vi "saveImage.vi"(9 "save_txt":bool, 10 "save_tiff":bool, 11 "image_info":T1={"file_path"=path "", "file_name"="", "image"=[], "image_size_xy"={"image_size_x_um"=1.0, "image_size_y_um"=1.0}, "pixel_dwell_time_ms"=1.0, "Laser_power_mW"=1.0, "pixel_size"=0.0, "tile_ij"={"tile_i"=0, "tile_j"=0}, "Objective"="", "ColorMarkers"=[], "timestamp"=timestamp(0 s since 1904-01-01), "micro-position-xyz"={"micro-position_x_mm"=1.0, "micro-position_y_mm"=1.0, "micro-position_z_mm"=1.0}, "zero_xyz"={"zero_x_mm"=0.0, "zero_y_mm"=0.0, "zero_z_mm"=0.0}, "nano-position-xyz"={"nano-position_x_V"=1.0, "nano-position_y_V"=1.0, "nano-position_z_V"=1.0}, "Kxyz"={"Kx_V/um"=1.0, "Ky_V/um"=1.0, "Kz_V/um"=1.0}}) -> ()   [LabVIEW 2018]
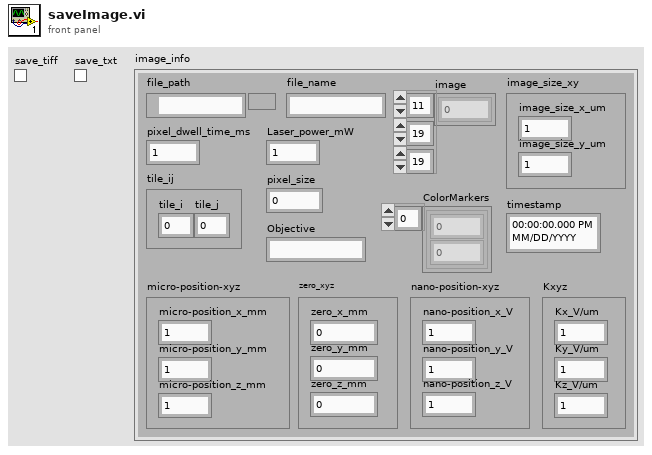
[diagram p1: front panel]
types:
  T1 = cluster{"file_path":path, "file_name":string, "image":dbl[][][], "image_size_xy":cluster{"image_size_x_um":sgl, "image_size_y_um":sgl}, "pixel_dwell_time_ms":sgl, "Laser_power_mW":sgl, "pixel_size":dbl, "tile_ij":cluster{"tile_i":i32, "tile_j":i32}, "Objective":string, "ColorMarkers":cluster{dbl, u32}[], "timestamp":timestamp, "micro-position-xyz":cluster{"micro-position_x_mm":sgl, "micro-position_y_mm":sgl, "micro-position_z_mm":sgl}, "zero_xyz":cluster{"zero_x_mm":dbl, "zero_y_mm":dbl, "zero_z_mm":dbl}, "nano-position-xyz":cluster{"nano-position_x_V":sgl, "nano-position_y_V":sgl, "nano-position_z_V":sgl}, "Kxyz":cluster{"Kx_V/um":sgl, "Ky_V/um":sgl, "Kz_V/um":sgl}}
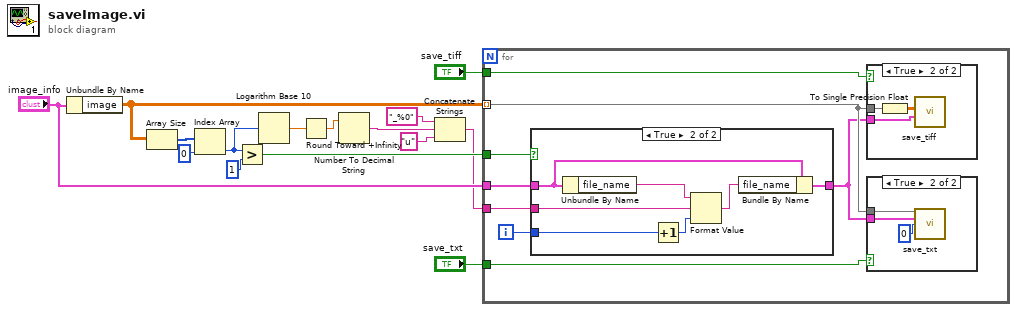
[diagram p0: block diagram]
diagram:
  n1 = Unbundle By Name("image_info") -> ("image"=w13:dbl[][][])
  n2 = Array Size(array=w13) -> (size(s)=w12:i32[])
  n3 = Index Array(array=w12, index=0) -> (element=w3:i32)
  n4 = Greater?(x=w3, y=1) -> (0:w9:bool)
  n5 = Logarithm Base 10(1:w3) -> (0:w2:dbl)
  n6 = Round Toward +Infinity(x=w2) -> (ceil(x): smallest int >= x=w1:dbl)
  n7 = Number To Decimal String(number=w1) -> (decimal integer string=w7:string)  [unwired: 1 in]
  n8 = Concatenate Strings("_%0" ("string"), w7, "u" ("string")) -> (w4:string)
  n9 = for {
    tunnel: "save_tiff" -> [w23]
    tunnel: "save_txt" -> [w22]
    tunnel: w13 -> [w21] mode=indexing
    tunnel: "image_info" -> [w18]
    tunnel: w9 -> [w20]
    tunnel: w4 -> [w16]
    i -> [w19]
    n10 = case shown="True" w20 {
      tunnel: w19 -> [_ w31]
      tunnel: w18 -> [w24 w26]
      tunnel: [w24 w28] -> w17
      tunnel: w16 -> [_ w25]
      frame False {
      }
      frame True {
        n11 = Unbundle By Name(w26) -> ("file_name"=w27:string)
        n12 = Increment(x=w31) -> (x+1=w30:i32)
        n13 = Format Value(string ("")=w27, format string=w25, value (0)=w30) -> (output string=w29:string)
        n14 = Bundle By Name(cluster=w26, "file_name"=w29) -> (w28:T1)
      }
    }
    n15 = case shown="True" w23 {
      tunnel: w21 -> [_ w35]
      tunnel: w17 -> [_ w37]
      frame False {
      }
      frame True {
        n16 = To Single Precision Float(number=w35) -> (single precision float=w36:sgl[][])
        n17 = call "save_tiff.vi"("image_info"=w37, "image_array"=w36) -> ()  [unwired: 10 in]
      }
    }
    n18 = case shown="True" w22 {
      tunnel: w21 -> [_ w34]
      tunnel: w17 -> [_ w33]
      frame False {
      }
      frame True {
        n19 = call "save_txt.vi"("image"=w34, "image_info"=w33, "run_number"=i16 0) -> ()  [unwired: 13 in]
      }
    }
  }
